vi "Create Scan SBlock.vi"(8 "error in (no error)":errorcluster, 11 "Schedule Block in":refnum<class "Schedule Block.lvclass">) -> (0 "error out":errorcluster, 3 "Scan SBlock out":refnum<class "Scan SBlock.lvclass">)   [LabVIEW 2020, in "Run Utilities.lvlib" / "Scan SBlock.lvclass"]
doc: "Create a new Scan SBlock from a Schedule Block"
uses:
  Scan SBlock.lvclass
  C:/Users/marco/Documents/GitHub_Lab/TALOS/talos/Run Utilities/Schedule Block/Schedule Block.lvclass
  Schedule Block/Schedule Block.lvclass
  Schedule/Schedule.lvclass
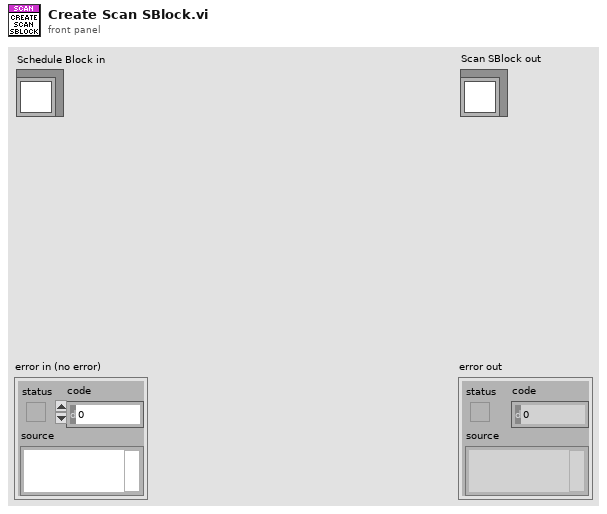
[diagram p1: front panel]
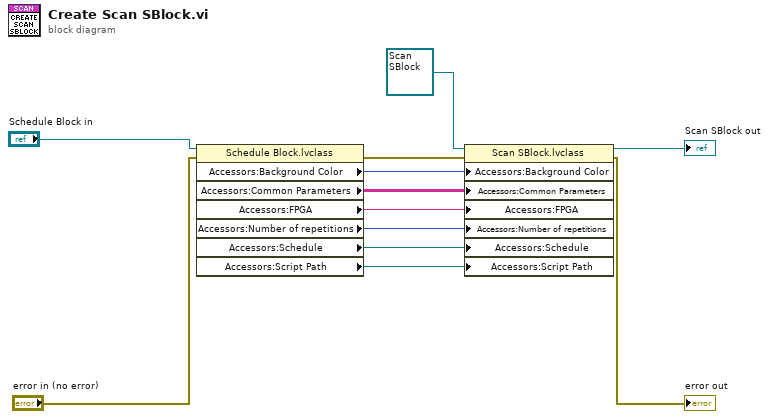
[diagram p0: block diagram]
diagram:
  n1 = property class="Schedule Block.lvclass"(reference="Schedule Block in", error in="error in (no error)") -> (error out=w9:errorcluster, "Accessors:Background Color"=w8:u32, "Accessors:Common Parameters"=w7:string[][], "Accessors:FPGA"=w6:string, "Accessors:Number of repetitions"=w5:u16, "Accessors:Schedule"=w4:refnum<class "Schedule.lvclass">, "Accessors:Script Path"=w3:path)  [unwired: 1 out]
  n2 = property class="Scan SBlock.lvclass"(reference=refnum<class "Scan SBlock.lvclass"> refnum ("Scan SBlock out"), error in=w9, "Accessors:Background Color"=w8, "Accessors:Common Parameters"=w7, "Accessors:FPGA"=w6, "Accessors:Number of repetitions"=w5, "Accessors:Schedule"=w4, "Accessors:Script Path"=w3) -> (reference out=→"Scan SBlock out":refnum<class "Scan SBlock.lvclass">, error out=→"error out":errorcluster)
